vi "Demo Scrolling.vi"(8 "error in (no error)":errorcluster) -> (0 "error out":errorcluster)   [LabVIEW 2011]
uses:
  VIremote.llb/VIremoteEvent.ctl
  VIremote.llb/VIremoteFunction.ctl
panel:
  in  "Radio Buttons":enum32{"Vertical", "Horizontal"}(radio)
  in  "String control":string="Tap me and I will scroll"
  in  "Slider":i32(slide)=21 scale=0.0..50.0
  in  "scroll back up":bool
  in  "scroll back":bool
  in  "VIremoteEvent":T1=enum."Connection Closed"
  # "Scrolling"
  # "If you make a panel larger than the screen on the device, you can enable scrolling. If the panel can't fit on your monitor then mouse emulation will not be used if a tap is made on a control that is not visible.\n\nNormal scroll is prefered for vertical scrolling to fill out forms or to display long texts.\n\nPage scroll is mostly used for horizontal scrolling. Each scroll will stop on multiples of the screen width. The page indicator can be used to display a dot for the current page.\n\nBoth horizontal and vertical scrolling at the same time should be avoided in most cases. \n\nUse buttons above to try out the most common scroll modes. This demo is not made for iPad."
  # "Notice the page indicator below. It can be placed at any vertical position. It will allways be centered horizontally."
  # "Scrolling"
  # "If sliders or other dragable objects are used in a scroll panel the user has to wait a second after touch down before the slider can be moved."
  # "Auto scroll enabled: If keyboard and mouse emulation is used then a control will be scrolled into view if it is hidden by the keyboard. This is true for the string control below."
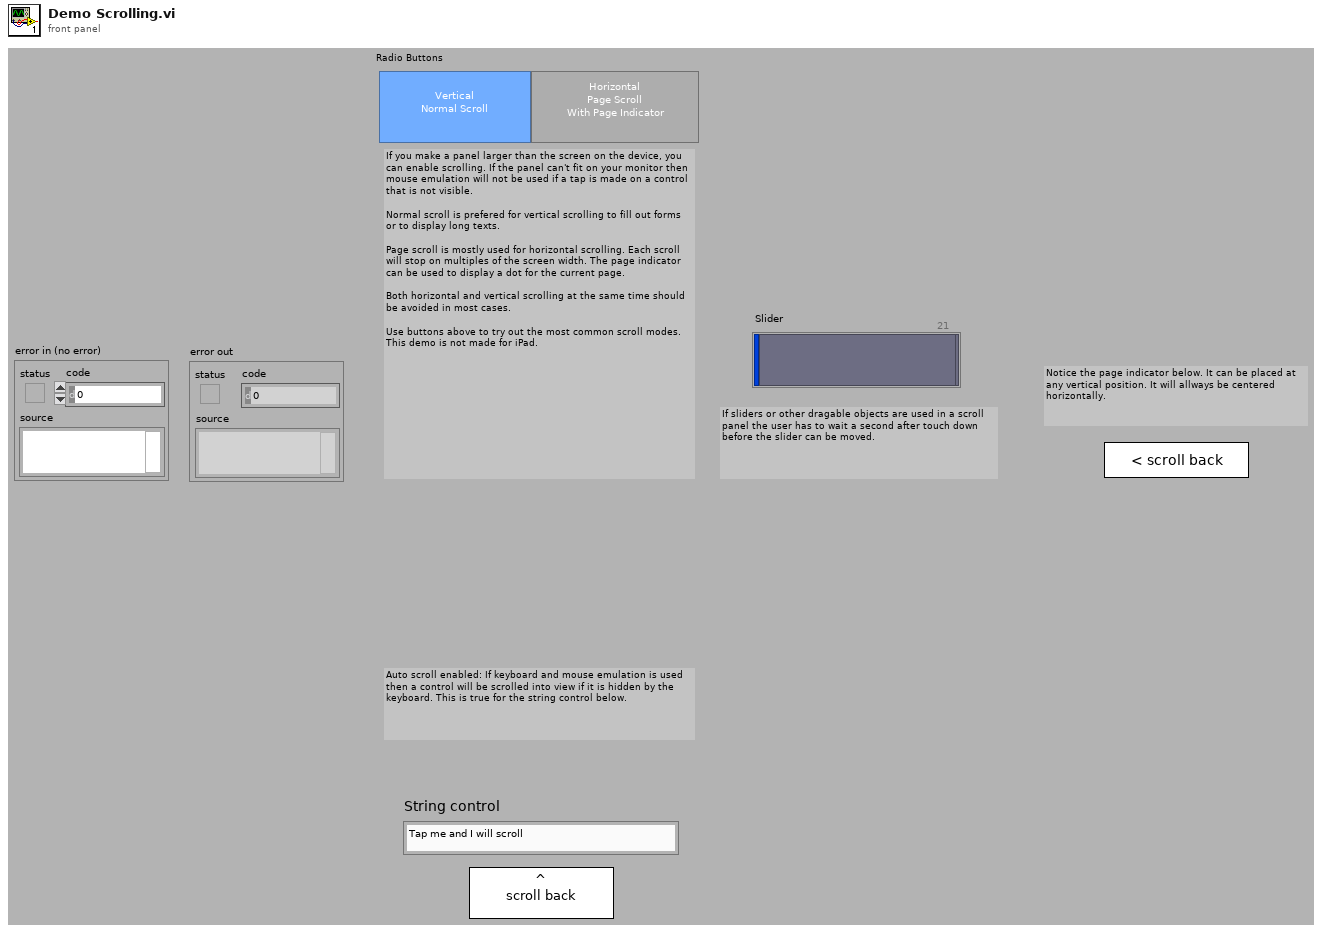
[diagram p1: front panel]
types:
  T1 = typedef "VIremoteEvent.ctl" = enum16{"No Event", "Connection Closed", "Navigate Back", "Enter Background", "Enter Foreground", "Portrait", "Portrait Upside Down", "Landscape Left", "Landscape Right"}
  T2 = typedef "VIremoteFunction.ctl" = enum16{"Do nothing", "Stop controller", "Close this connection", "Show info panel", "Set VI to control", "Set Accelerometer freq (Hz)", "Show Alert message", "Start Sound Input", "Stop Sound Input", "Set Volume (0-100)", "Set sound output Speaker", "Set sound output Receiver", "Play Sound", "Repeat Sound", "Stop Sound", "Pause Sound", "Resume Sound", "Set panel width of caller (320 or 480)", "Set Panel Size to Portrait", "Set Panel Size to Landscape", "Set Panel Size as Current Orientation", "Allow all UI Orientations", "Send user notification", "Disable Scrolling", "Normal Scrolling", "Page Scrolling", "Set Scroll Offset", "Page Indicator Position"}
  T3 = typedef "LVRectTypeDef.ctl" = cluster{"left":i16, "top":i16, "right":i16, "bottom":i16}
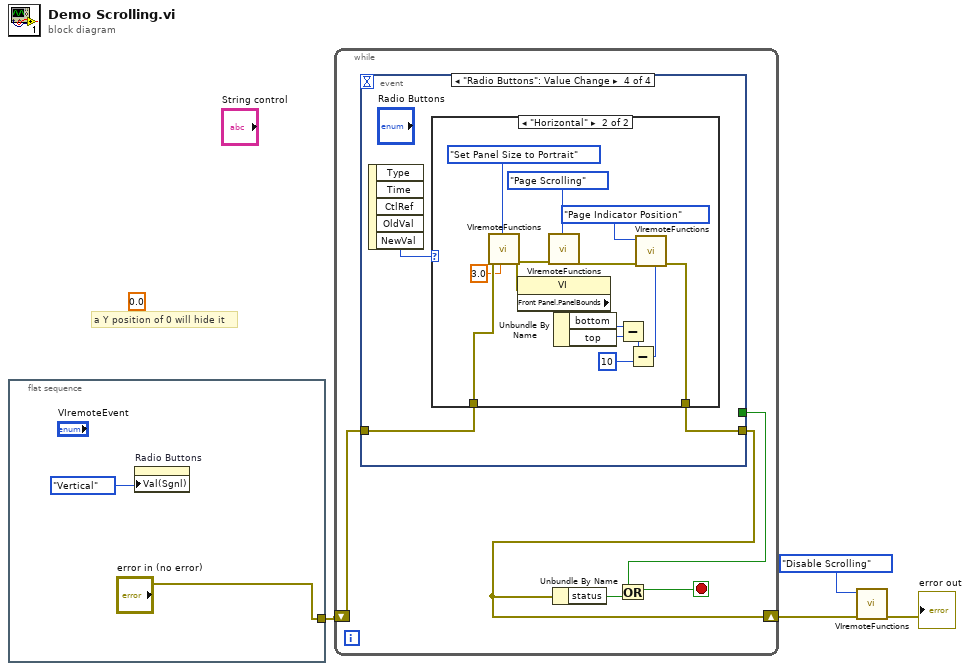
[diagram p0: block diagram]
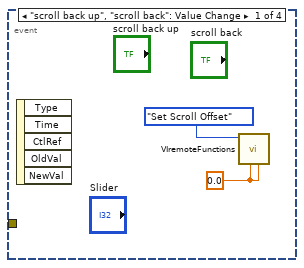
[diagram p2: hidden frame]
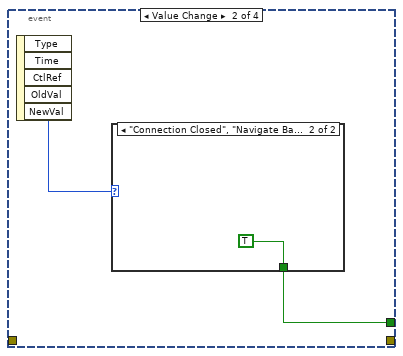
[diagram p3: hidden frame]
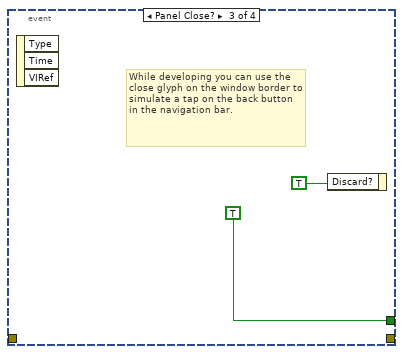
[diagram p5: hidden frame]
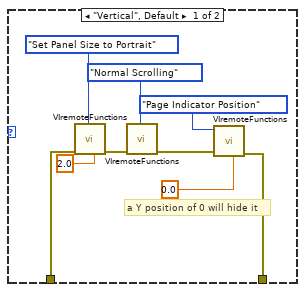
[diagram p6: hidden frame]
diagram:
  (unwired) 0.0 ("Value in Y")
  # "a Y position of 0 will hide it"
  n1 = flat-sequence {
    tunnel: ["error in (no error)"] -> w4
    frame #0 {
      n2 = property on="Radio Buttons" class="RadioBtnsControl (strict)"("Val(Sgnl)"=enum32{"Vertical", "Horizontal"}."Vertical" ("Radio Buttons")) -> ()  [unwired: 2 in, 2 out]
    }
  }
  n3 = while {
    shift-right: [w8] -> w2
    shift-left: w4 -> [w9]
    stop <- w11 stop-if-true
    n4 = event shown="[3] \"Radio Buttons\": Value Change" {
      selector: _ -> [_ _ _ _]
      dyn-events: _ -> [_ _ _ _]
      timeout: _ -> [_ _ _ _]
      tunnel: [_ _ _ w19] -> w8
      tunnel: w9 -> [_ _ _ w20]
      tunnel: [_ w14 TRUE ("Discard?") _] -> w7
      event "scroll back up", "scroll back": Value Change {
        w12 = 0.0 ("Value in")
        n5 = event-data() -> ()  [unwired: 6 out]
        n6 = call "VIremoteFunctions.vi"("Value in Y"=w12, "Value in X"=w12, "Function"=VIremoteFunction."Set Scroll Offset") -> ()  [unwired: 3 in, 6 out]
      }
      event Value Change {
        n7 = event-data() -> ("NewVal"=w15:T1)  [unwired: 5 out]
        n8 = case shown="\"Connection Closed\", \"Navigate Back\"" w15 {
          tunnel: [_ TRUE] -> w14
          frame "No Event", Default {
          }
          frame "Connection Closed", "Navigate Back" {
          }
        }
      }
      event Panel Close? {
        # "While developing you can use the close glyph on the window border to simulate a tap on the back button in the navigation bar."
        n9 = event-data() -> ()  [unwired: 4 out]
        n10 = event-data("Discard?"=TRUE) -> ()  [unwired: 1 in, 1 out]
      }
      event "Radio Buttons": Value Change {
        n11 = event-data() -> ("NewVal"=w21:enum32{"Vertical", "Horizontal"})  [unwired: 5 out]
        n12 = case shown="\"Horizontal\"" w21 {
          tunnel: w20 -> [w23 w34]
          tunnel: [w22 w31] -> w19
          frame "Vertical", Default {
            # "a Y position of 0 will hide it"
            n13 = call "VIremoteFunctions.vi"("Value in Y"=2.0, "error in (no error)"=w23, "Function"=VIremoteFunction."Set Panel Size to Portrait") -> ("error out"=w26:errorcluster)  [unwired: 3 in, 5 out]
            n14 = call "VIremoteFunctions.vi"("error in (no error)"=w26, "Function"=VIremoteFunction."Normal Scrolling") -> ("error out"=w25:errorcluster)  [unwired: 4 in, 5 out]
            n15 = call "VIremoteFunctions.vi"("Value in Y"=0.0, "error in (no error)"=w25, "Function"=VIremoteFunction."Page Indicator Position") -> ("error out"=w22:errorcluster)  [unwired: 3 in, 5 out]
          }
          frame "Horizontal" {
            n16 = call "VIremoteFunctions.vi"("Value in X"=3.0 ("Value in Y"), "error in (no error)"=w34, "Function"=VIremoteFunction."Set Panel Size to Portrait") -> ("error out"=w32:errorcluster)  [unwired: 3 in, 5 out]
            n17 = property class="VI"(error in=w32) -> ("Front Panel.PanelBounds"=w41:T3)  [unwired: 1 in, 2 out]
            n18 = call "VIremoteFunctions.vi"("error in (no error)"=w32, "Function"=VIremoteFunction."Page Scrolling") -> ("error out"=w36:errorcluster)  [unwired: 4 in, 5 out]
            n19 = Unbundle By Name(w41) -> ("bottom"=w40:i16, "top"=w39:i16)
            n20 = Subtract(x=w40, y=w39) -> (x-y=w42:i16)
            n21 = Subtract(x=w42, y=i16 10) -> (x-y=w38:i16)
            n22 = call "VIremoteFunctions.vi"("Value in Y"=w38, "error in (no error)"=w36, "Function"=VIremoteFunction."Page Indicator Position") -> ("error out"=w31:errorcluster)  [unwired: 3 in, 5 out]
          }
        }
      }
    }
    n23 = Unbundle By Name(w8) -> ("status"=w10:bool)
    n24 = Or(x=w7, y=w10) -> (x .or. y?=w11:bool)
  }
  n25 = call "VIremoteFunctions.vi"("error in (no error)"=w2, "Function"=VIremoteFunction."Disable Scrolling") -> ("error out"=→"error out":errorcluster)  [unwired: 4 in, 5 out]
